vi "Add Network Resource.vi"(8 "error in (no error)":errorcluster, 9 "local name for device":string, 10 "password":string, 11 "name of network device":string) -> (0 "error out":errorcluster)   [LabVIEW 2020, in "MacroAssert.lvlib" / "WINNET.lvlib"]
doc: "This VI will connect a network drive or printer to a local device (e.g. F: or LPT3). The network name is the UNC name of the network resource. For example, if LabVIEW was installed on a shared network volume with a machine name of APPLICATIONS, on which the LabVIEW directory resided in a directory called WINAPPS, the UNC name for the \"name of network device\" would be: \\\\APPLICATIONS\\WINAPPSS\\LABVIEW"
uses:
  WINNET.lvlib
  MPR.DLL
panel:
  out "error codes":string="WN_SUCCESS                         0x0000 Function was successful.\nWN_NOT_SUPPORTED         0x0001 Function was not supported.\nWN_NET_ERROR                   0x0002 An error occurred on the network.\nWN_BAD_POINTER                0x0004 The pointer was invalid.\nWN_BAD_PASSWORD           0x0006 The password was invalid.\nWN_ACCESS_DENIED            0x0007 A security violation occurred.\nWN_OUT_OF_MEMORY          0x000B The system was out of memory.\nWN_BAD_LOCALNAME           0x0033 The local device name was invalid.\nWN_ALREADY_CONNECTED 0x0034 The local device was already connected to a remote resource."
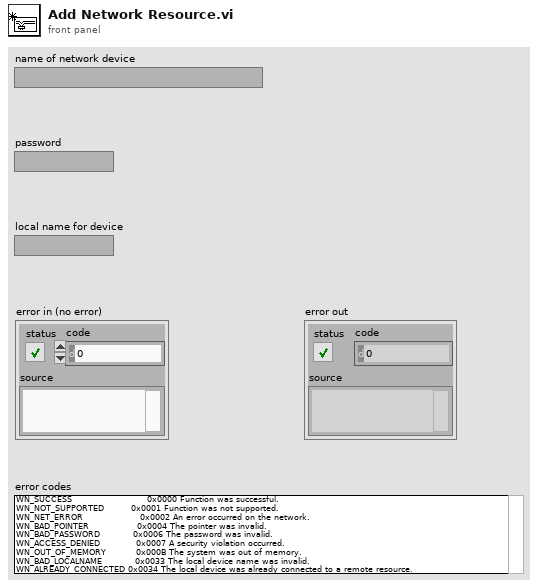
[diagram p1: front panel]
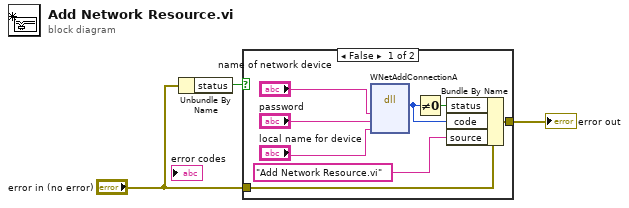
[diagram p0: block diagram]
diagram:
  n1 = Unbundle By Name("error in (no error)") -> ("status"=w3:bool)
  n2 = case shown="False" w3 {
    tunnel: "error in (no error)" -> [w7 w12]
    tunnel: [w6 w12] -> w1
    frame False {
      n3 = dll-call lib="MPR.DLL" fn="WNetAddConnectionA"("lpszNetPath"="name of network device", "lpszPassword"="password", "lpszLocalName"="local name for device") -> ("ReturnVal"=w9:u32)  [unwired: 6 in, 2 out]
      n4 = Not Equal To 0?(x=w9) -> (x != 0?=w10:bool)
      n5 = Bundle By Name(cluster=w7, "status"=w10, "code"=w9, "source"="Add Network Resource.vi") -> (w6:errorcluster)
    }
    frame True {
    }
  }
  "error out" <- w1
